vi "Execute Test Vector.vi"(8 "error in (no error)":errorcluster, 11 "LUnit Test Vector in":refnum<class "LUnit Test Vector.lvclass">) -> (0 "error out":errorcluster, 3 "LUnit Test Vector out":refnum<class "LUnit Test Vector.lvclass">)   [LabVIEW 2020, in "LUnit Test Vector.lvclass"]
doc: "This VI executes the configured test vector components. The vector must be setup with at least one component and a VI under test before executing this VI."
uses:
  LUnit Test Vector.lvclass
  Test Case/LUnit Test Case.lvclass
  C:/Users/anton/Documents/GitHub/LUnit/source/Framework/Test Case/LUnit Test Case.lvclass
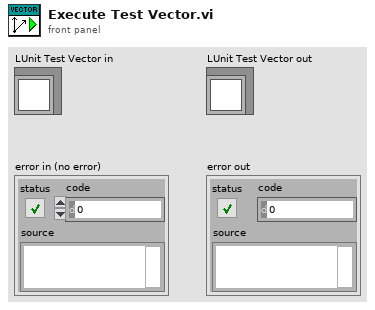
[diagram p1: front panel]
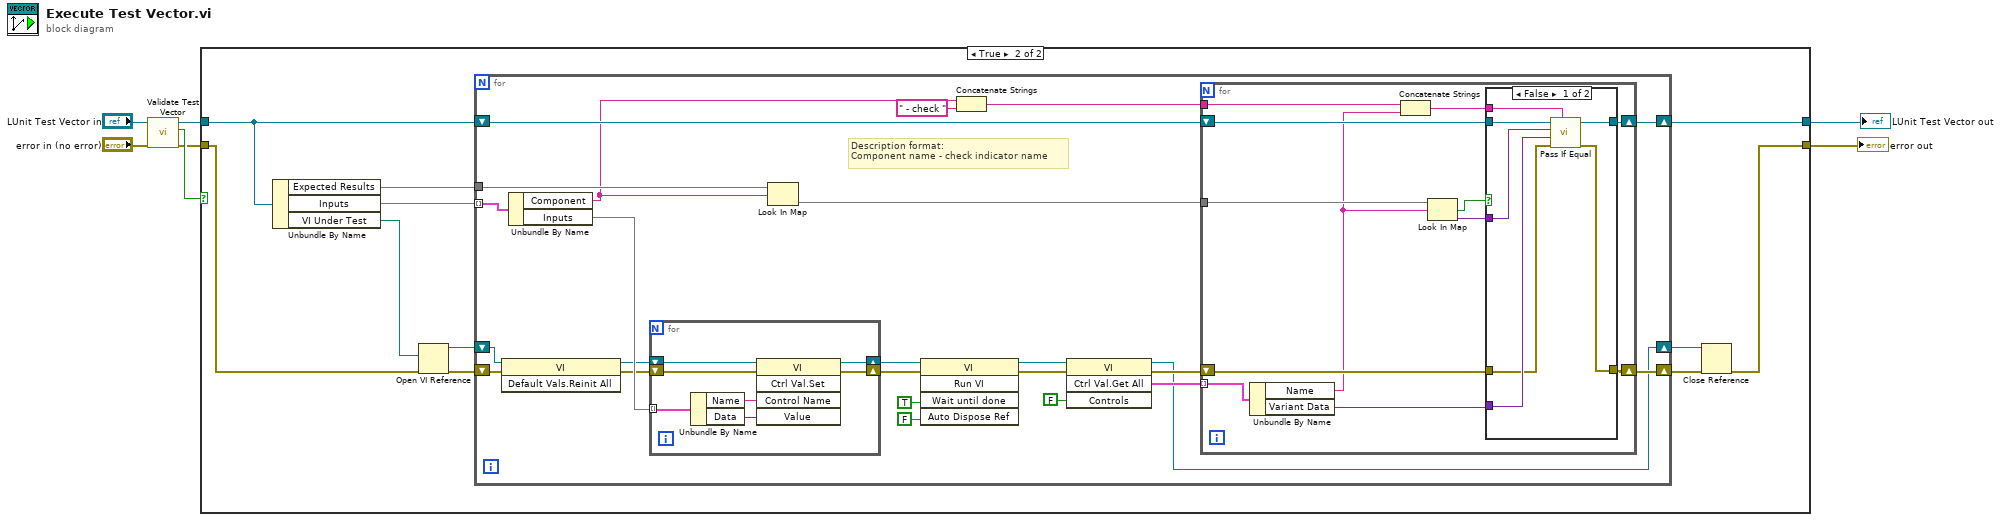
[diagram p0: block diagram]
diagram:
  n1 = call "Validate Test Vector.vi"("error in (no error)"="error in (no error)", "LUnit Test Vector in"="LUnit Test Vector in") -> ("error out"=w5:errorcluster, "Valid?"=w7:bool, "LUnit Test Vector out"=w2:refnum<class "LUnit Test Vector.lvclass">)  [unwired: 7 in]
  n2 = case shown="True" w7 {
    tunnel: w2 -> [w9 w18]
    tunnel: [w9 w17] -> w3
    tunnel: [w8 w10] -> w4
    tunnel: w5 -> [w8 w16]
    frame False {
    }
    frame True {
      n3 = Unbundle By Name(w18) -> ("Expected Results"=w20:map{string, map{string, variant}}, "Inputs"=w19:map{string, map{string, variant}}, "VI Under Test"=w15:path)
      n4 = Open VI Reference(vi path=w15, error in (no error)=w16) -> (vi reference=w13:refnum<vi>, error out=w14:errorcluster)  [unwired: 4 in]
      n5 = for {
        tunnel: w19 -> [w38] mode=indexing
        shift-right: [w34] -> w17
        shift-left: w18 -> [w36]
        tunnel: w20 -> [w31]
        shift-right: [w33] -> w11
        shift-left: w14 -> [w27]
        shift-right: [w24] -> w12
        shift-left: w13 -> [w28]
        # "Description format:\nComponent name - check indicator name"
        n6 = invoke class="VI" method="Default Vals.Reinit All"(reference=w28, error in=w27) -> (reference out=w26:refnum<vi>, error out=w25:errorcluster)  [unwired: 1 in, 1 out]
        n7 = Unbundle By Name(w38) -> ("Component"=w23:string, "Inputs"=w37:map{string, variant})
        n8 = for {
          shift-right: [w49] -> w42
          shift-left: w26 -> [w51]
          shift-right: [w48] -> w41
          shift-left: w25 -> [w50]
          tunnel: w37 -> [w47] mode=indexing
          n9 = Unbundle By Name(w47) -> ("Name"=w46:string, "Data"=w45:variant)
          n10 = invoke class="VI" method="Ctrl Val.Set"(reference=w51, error in=w50, "Control Name"=w46, "Value"=w45) -> (reference out=w49:refnum<vi>, error out=w48:errorcluster)  [unwired: 1 in, 3 out]
        }
        n11 = Look In Map(map=w31, key=w23) -> (value=w30:map{string, variant})  [unwired: 1 in, 1 out]
        n12 = invoke class="VI" method="Run VI"(reference=w42, error in=w41, "Wait until done"=TRUE ("Wait Until Done"), "Auto Dispose Ref"=FALSE ("Auto Dispose Reference")) -> (reference out=w29:refnum<vi>, error out=w40:errorcluster)  [unwired: 1 in, 3 out]
        n13 = Concatenate Strings(w23, " - check " ("string")) -> (w21:string)
        n14 = invoke class="VI" method="Ctrl Val.Get All"(reference=w29, error in=w40, "Controls"=FALSE) -> (reference out=w24:refnum<vi>, error out=w32:errorcluster, "Get All Control Values Variant"=w35:cluster{"Name":string, "Variant Data":variant}[])  [unwired: 1 in, 1 out]
        n15 = for {
          tunnel: w35 -> [w63] mode=indexing
          tunnel: w30 -> [w62]
          shift-right: [w61] -> w34
          shift-left: w36 -> [w60]
          shift-right: [w57] -> w33
          shift-left: w32 -> [w56]
          tunnel: w21 -> [w52]
          n16 = Unbundle By Name(w63) -> ("Name"=w55:string, "Variant Data"=w58:variant)
          n17 = Concatenate Strings(w52, w55) -> (w53:string)
          n18 = Look In Map(map=w62, key=w55) -> (key not found?=w54:bool, value=w59:variant)  [unwired: 1 in]
          n19 = case shown="False" w54 {
            tunnel: [w70 w72] -> w61
            tunnel: w60 -> [w69 w72]
            tunnel: w59 -> [w68 _]
            tunnel: w58 -> [w67 _]
            tunnel: [w66 w71] -> w57
            tunnel: w56 -> [w65 w71]
            tunnel: w53 -> [w64 _]
            frame False {
              n20 = call "Pass If Equal.vi"("Description"=w64, "error in (no error)"=w65, "Actual"=w67, "Expected"=w68, "LUnit Test Case In"=w69) -> ("error out"=w66:errorcluster, "LUnit Test Case Out"=w70:refnum<class "LUnit Test Vector.lvclass">)  [unwired: 5 in]
            }
            frame True {
              # "Ignore output"
            }
          }
        }
      }
      n21 = Close Reference(reference=w12, error in (no error)=w11) -> (error out=w10:errorcluster)
    }
  }
  "error out" <- w4
  "LUnit Test Vector out" <- w3
